vi "Match Cluster to CSV.vi"(11 "Match Cluster":T1) -> ()   [LabVIEW 2015]
uses:
  <vilib>/Utility/file.llb/Write Delimited Spreadsheet (string).vi
panel:
  in  "output csv":path=path "C:/Users/a0272913/Desktop/AppRawJSON/output4.csv"
  in  "path to png file":path=path "C:/Users/a0272913/Desktop/AppRawJSON/drawing.png"
  out "2D Picture":picture
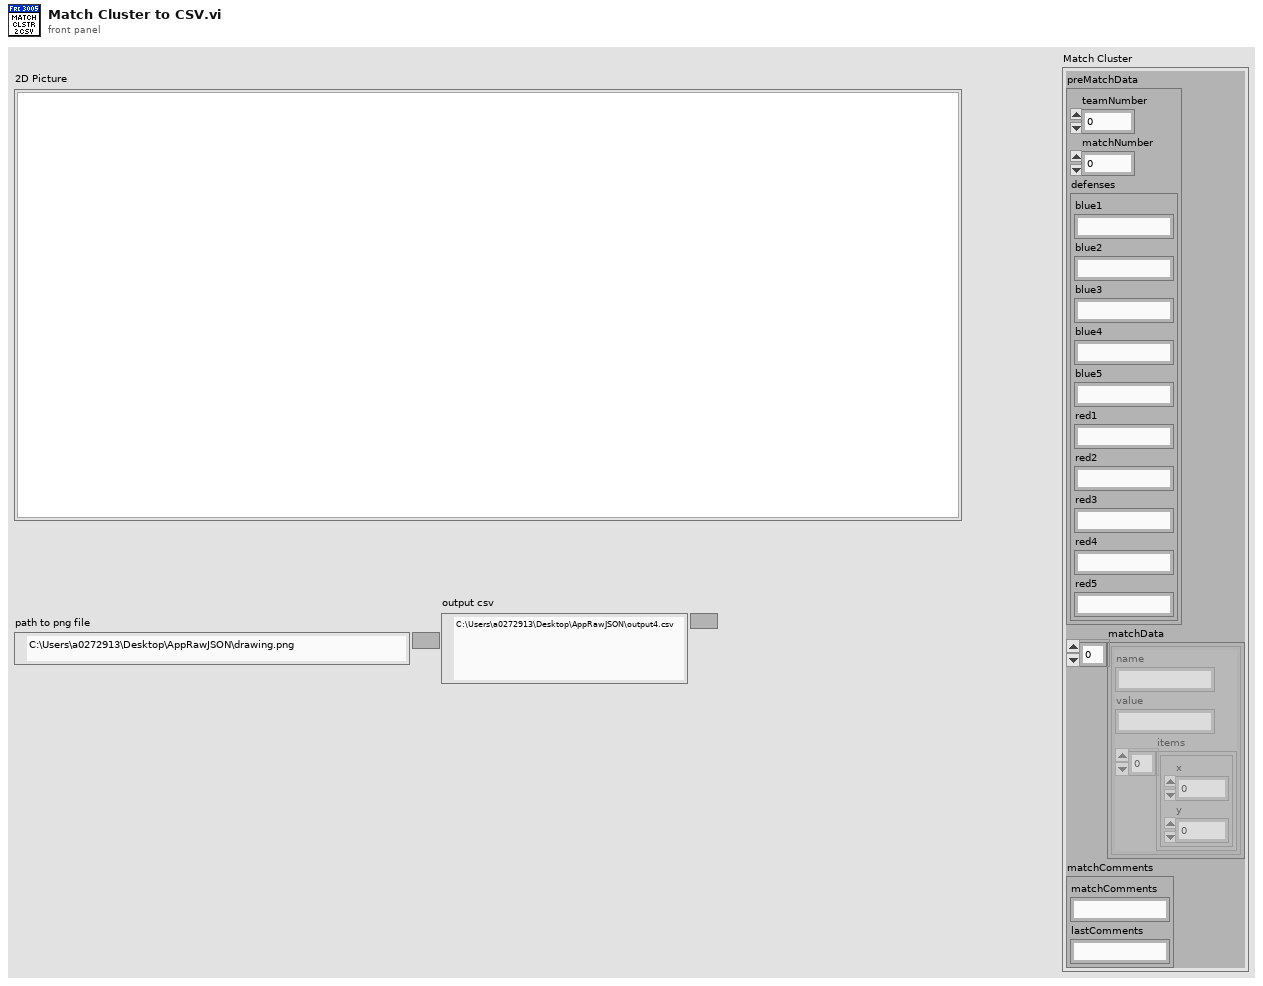
[diagram p1: front panel]
types:
  T1 = typedef "JSONCluster.ctl" = cluster{"preMatchData":cluster{"teamNumber":i32, "matchNumber":i32, "defenses":cluster{"blue1":string, "blue2":string, "blue3":string, "blue4":string, "blue5":string, "red1":string, "red2":string, "red3":string, "red4":string, "red5":string}}, "matchData":cluster{"name":string, "value":string, "items":cluster{"x":i32, "y":i32}[]}[], "matchComments":cluster{"matchComments":string, "lastComments":string}}
  T2 = typedef "LVBoundsTypeDef.ctl" = cluster{"Width":u32, "Height":u32}
  T3 = cluster{"teamNumber":i32, "matchNumber":i32, "defenses":cluster{"blue1":string, "blue2":string, "blue3":string, "blue4":string, "blue5":string, "red1":string, "red2":string, "red3":string, "red4":string, "red5":string}}
  T4 = cluster{"name":string, "value":string, "items":cluster{"x":i32, "y":i32}[]}[]
  T5 = typedef "imagedata.ctl" = cluster{"image type":i32, "image depth":i32, "image":u8[], "mask":u8[], "colors":u32[], "Rectangle":cluster{"left":i16, "top":i16, "right":i16, "bottom":i16}}
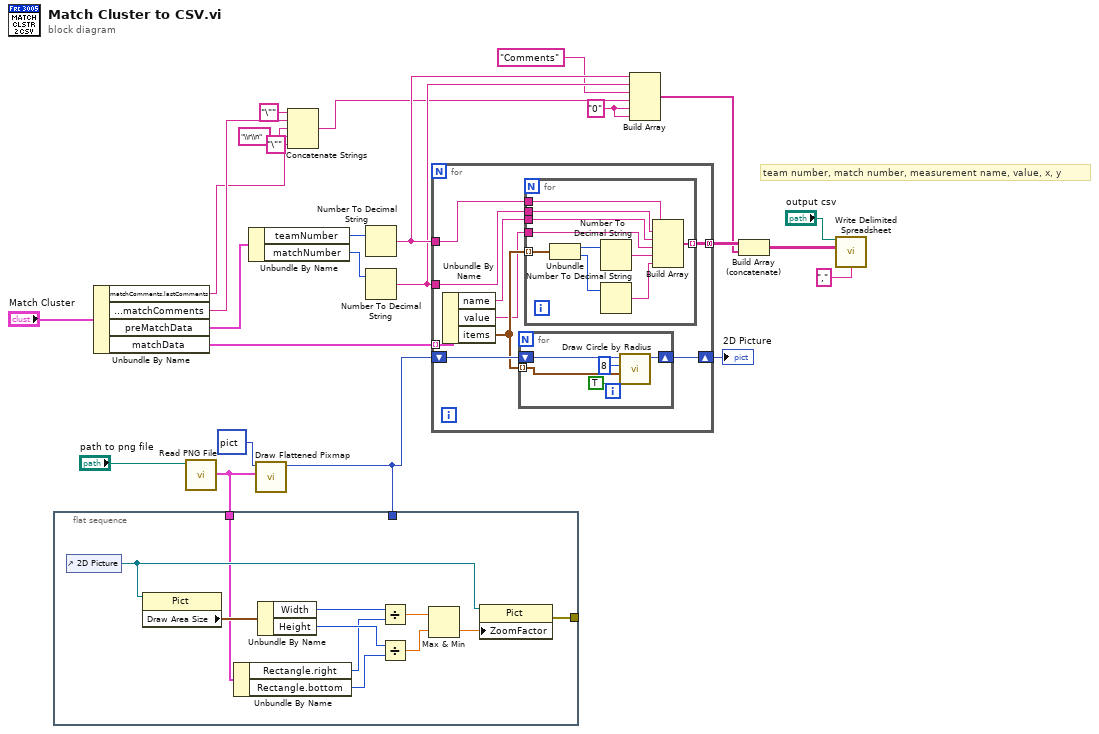
[diagram p0: block diagram]
diagram:
  w8 = "0" ("element")
  # "team number, match number, measurement name, value, x, y"
  n1 = flat-sequence {
    tunnel: w24 -> [w27]
    tunnel: [w26] -> _
    tunnel: w18 -> [_]
    frame #0 {
      n2 = control-ref of="2D Picture"() -> (w28:refnum<vi>)
      n3 = property class="Pict"(reference=w28) -> ("Draw Area Size"=w33:T2)  [unwired: 1 in, 2 out]
      n4 = Unbundle By Name(w27) -> ("Rectangle.right"=w30:i16, "Rectangle.bottom"=w29:i16)
      n5 = Unbundle By Name(w33) -> ("Width"=w32:u32, "Height"=w31:u32)
      n6 = Divide(x=w32, y=w30) -> (x/y=w34:dbl)
      n7 = Divide(x=w31, y=w29) -> (x/y=w35:dbl)
      n8 = Max & Min(x=w34, y=w35) -> (min(x,y)=w36:dbl)  [unwired: 1 out]
      n9 = property class="Pict"(reference=w28, "ZoomFactor"=w36) -> (error out=w26:errorcluster)  [unwired: 1 in, 1 out]
    }
  }
  n10 = Unbundle By Name("Match Cluster") -> ("matchComments.lastComments"=w10:string, "matchComments.matchComments"=w11:string, "preMatchData"=w19:T3, "matchData"=w22:T4)
  n11 = call <vilib>:"Read PNG File.vi"("path to PNG file"="path to png file") -> ("image data"=w24:T5)  [unwired: 8 in, 2 out]
  n12 = Unbundle By Name(w19) -> ("teamNumber"=w17:i32, "matchNumber"=w16:i32)
  n13 = call <vilib>:"Draw Flattened Pixmap.vi"("image data"=w24, "picture"=picture data[5B]) -> ("new picture"=w18:picture)  [unwired: 7 in]
  n14 = Concatenate Strings("\"" ("string"), w11, "\\r\\n" ("string"), w10, "\"" ("string")) -> (w9:string)
  n15 = Number To Decimal String(number=w17) -> (decimal integer string=w15:string)  [unwired: 1 in]
  n16 = Number To Decimal String(number=w16) -> (decimal integer string=w14:string)  [unwired: 1 in]
  n17 = for {
    shift-right: [w44] -> w23
    shift-left: w18 -> [w45]
    tunnel: w22 -> [w43] mode=indexing
    tunnel: w15 -> [w39]
    tunnel: w14 -> [w38]
    tunnel: [w37] -> w7 mode=concatenating
    n18 = Unbundle By Name(w43) -> ("name"=w41:string, "value"=w40:string, "items"=w42:cluster{"x":i32, "y":i32}[])
    n19 = for {
      shift-right: [w59] -> w44
      shift-left: w45 -> [w60]
      tunnel: w42 -> [w58] mode=indexing
      n20 = call <vilib>:"Draw Circle by Radius.vi"("fill?(F)"=TRUE, "pixel center"=w58, "radius"=i16 8, "picture"=w60) -> ("new picture"=w59:picture)  [unwired: 7 in]
    }
    n21 = for {
      tunnel: w42 -> [w55] mode=indexing
      tunnel: w41 -> [w49]
      tunnel: w40 -> [w50]
      tunnel: w39 -> [w48]
      tunnel: w38 -> [w47]
      tunnel: [w46] -> w37 mode=indexing
      n22 = Unbundle(w55) -> ("x"=w54:i32, "y"=w53:i32)
      n23 = Number To Decimal String(number=w54) -> (decimal integer string=w51:string)  [unwired: 1 in]
      n24 = Number To Decimal String(number=w53) -> (decimal integer string=w52:string)  [unwired: 1 in]
      n25 = Build Array(w48, w47, w49, w50, w51, w52) -> (w46:string[])
    }
  }
  "2D Picture" <- w23
  n26 = Build Array(w15, w14, "Comments" ("element"), w9, w8, w8) -> (w6:string[])
  n27 = Build Array (concatenate)(w7, w6) -> (w5:string[][])
  n28 = call-poly <vilib>:"Write Delimited Spreadsheet.vi"("file path (dialog if empty)"="output csv", "2D data"=w5, "delimiter (\\t)"="," ("delimiter (\\t)")) -> ()  [unwired: 11 in, 2 out]
